vi "Queue Status.vi"(8 "error in":errorcluster, 11 "QueueMessageTransport in":refnum<class "QueueMessageTransport.lvclass">) -> (0 "error out":errorcluster, 2 "Queue Status":T1, 3 "QueueMessageTransport out":refnum<class "QueueMessageTransport.lvclass">)   [LabVIEW 2016, in "QueueMessageTransport.lvclass"]
uses:
  QueueMessageTransport.lvclass
  _Typedefs/Queue Status.ctl
  QueueMessageTransport.lvclass/QueueMessageTransport.ctl
  IMessagePayload/IMessagePayload.lvclass
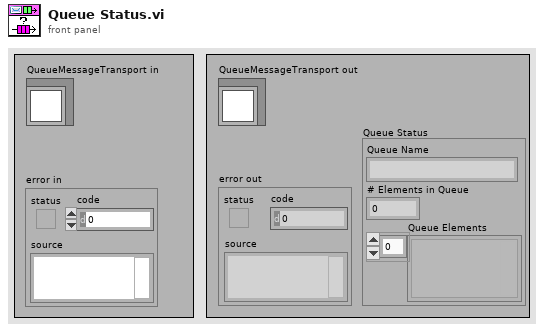
[diagram p1: front panel]
types:
  T1 = typedef "QueueMessageTransport.lvclass/Queue Status.ctl" = cluster{"Queue Name":string, "# Elements in Queue":i32, "Queue Elements":variant[]}
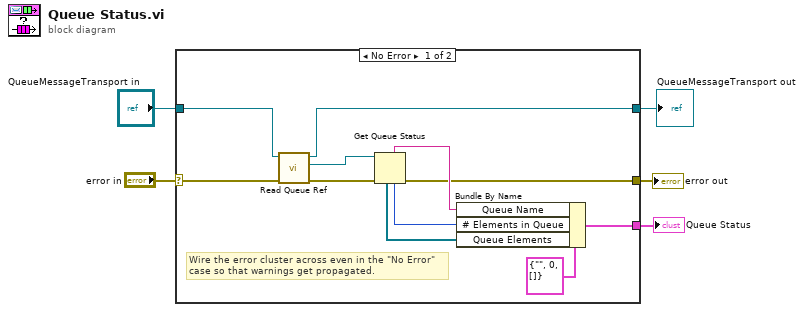
[diagram p0: block diagram]
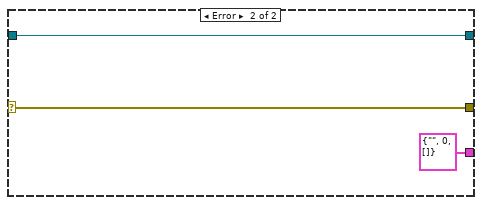
[diagram p2: hidden frame]
diagram:
  n1 = case shown="No Error" "error in" {
    selector: "error in" -> [w16 w19]
    tunnel: [w6 w19] -> w4
    tunnel: [w14 w18] -> w2
    tunnel: "QueueMessageTransport in" -> [w15 w18]
    tunnel: [w11 T1 {"Queue Name"="", "# Elements in Queue"=0, "Queue Elements"=[]} ("Queue Status")] -> w1
    frame No Error {
      # "Wire the error cluster across even in the \"No Error\"\ncase so that warnings get propagated."
      n2 = call "Read Queue Ref.vi"("error in"=w16, "QueueMessageTransport in"=w15) -> ("error out"=w13:errorcluster, "Queue Ref"=w12:refnum<queue>, "QueueMessageTransport out"=w14:refnum<class "QueueMessageTransport.lvclass">)  [unwired: 7 in]
      n3 = Get Queue Status(queue=w12, error in (no error)=w13) -> (queue name=w9:string, error out=w6:errorcluster, # elements in queue=w8:i32, elements=w7:refnum<class "IMessagePayload.lvclass">[])  [unwired: 1 in, 4 out]
      n4 = Bundle By Name(cluster=T1 {"Queue Name"="", "# Elements in Queue"=0, "Queue Elements"=[]} ("Queue Status"), "Queue Name"=w9, "# Elements in Queue"=w8, "Queue Elements"=w7) -> (w11:T1)
    }
    frame Error {
    }
  }
  "error out" <- w4
  "QueueMessageTransport out" <- w2
  "Queue Status" <- w1
